vi "Test SQL.vi"() -> ()   [LabVIEW 2020]
uses:
  <vilib>/addons/database/NI_Database_API.lvlib
  <vilib>/addons/database/Connection.llb/DB Tools Open Connec (Path).vi
  <vilib>/addons/database/Connection.llb/Conn Execute.vi
  <vilib>/addons/database/Recordset.llb/Rec Fetch Recordset Data (R).vi
  <vilib>/addons/database/Recordset.llb/Rec Destroy - Connection.vi
panel:
  out "recordset data":variant[][](array[variant])
  out "error out":errorcluster
  in  "connection information":path
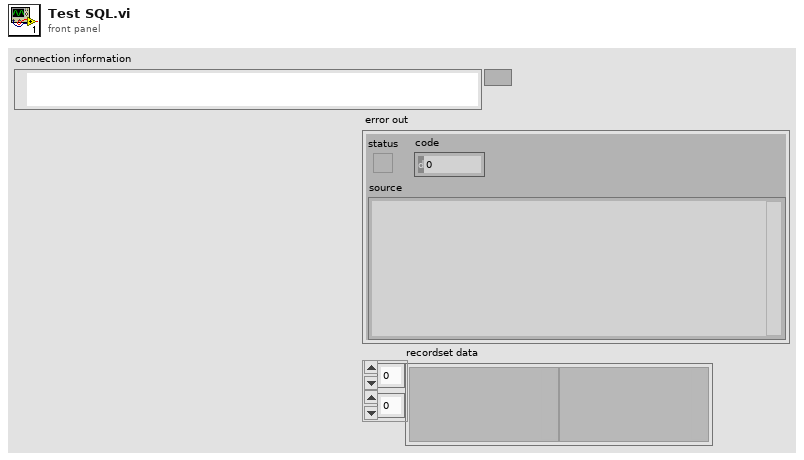
[diagram p1: front panel]
types:
  T1 = typedef "NI_Database_API.lvlib/Conn ObjectReference.ctl" = refnum<k1>
  T2 = typedef "NI_Database_API.lvlib/Rec ObjectReference.ctl" = refnum<k1>
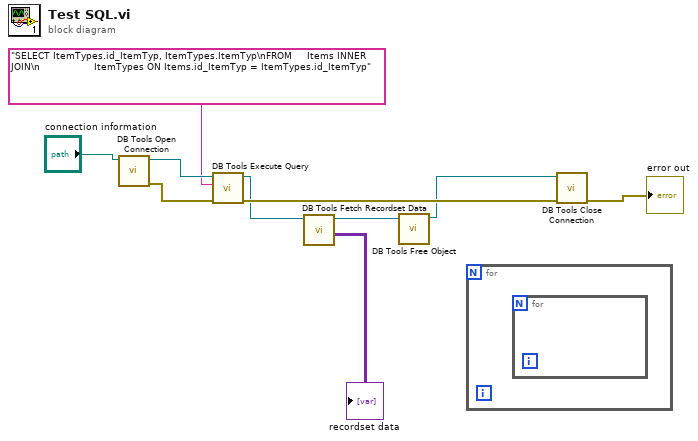
[diagram p0: block diagram]
diagram:
  n1 = call-poly <vilib>:"DB Tools Open Connection.vi"("connection information"="connection information") -> ("error out"=w7:errorcluster, "connection reference"=w8:T1)  [unwired: 7 in]
  n2 = call-poly <vilib>:"DB Tools Execute Query.vi"("error in (no error)"=w7, "SQL query"="SELECT ItemTypes.id_ItemTyp, ItemTypes.ItemTyp\nFROM     Items INNER JOIN\n                  ItemTypes ON Items.id_ItemTyp = ItemTypes.id_ItemTyp", "connection reference"=w8) -> ("error out"=w6:errorcluster, "recordset reference"=w4:T2)  [unwired: 5 in]
  n3 = call-poly <vilib>:"DB Tools Fetch Recordset Data.vi"("recordset reference"=w4) -> ("recordset data"=→"recordset data":variant[][], "recordset reference out"=w2:T2)  [unwired: 4 in, 1 out]
  n4 = call-poly <vilib>:"DB Tools Free Object.vi"("recordset reference"=w2) -> ("connection reference"=w1:T1)  [unwired: 9 in, 1 out]
  n5 = for {
    n6 = for {
    }
  }
  n7 = call <vilib>:"DB Tools Close Connection.vi"("error in (no error)"=w6, "connection reference"=w1) -> ("error out"=→"error out":errorcluster)  [unwired: 5 in]
